vi "Add DefinedName.vi"(7 "Sheet Name":string, 8 "error in":errorcluster, 9 "Cell Range":string, 10 "Identifier":string, 11 "SpreadsheetDoc in":refnum<k24>) -> (0 "error out":errorcluster, 3 "SpreadsheetDoc out":refnum<k24>)   [LabVIEW 2019, in "Open Xml.lvlib"]
uses:
  Open Xml.lvlib
  D:/git/Open-Xml-LabVIEW/Source/DocumentFormat.OpenXml.dll
  DocumentFormat.OpenXml.dll
  D:/git/Open-Xml-LabVIEW/Source/DocumentFormat.OpenXml.Framework.dll
  DocumentFormat.OpenXml.Framework.dll
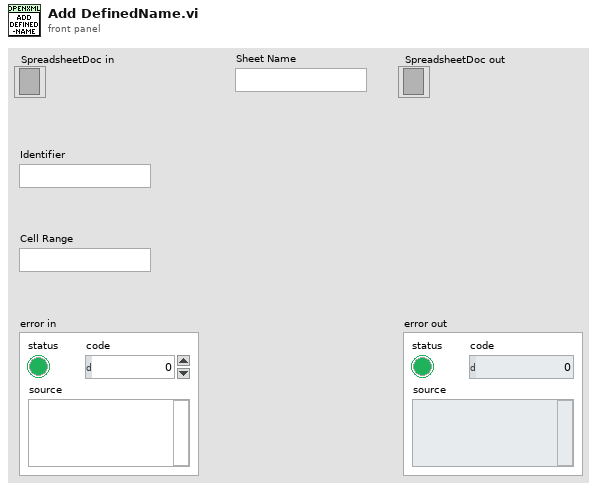
[diagram p1: front panel]
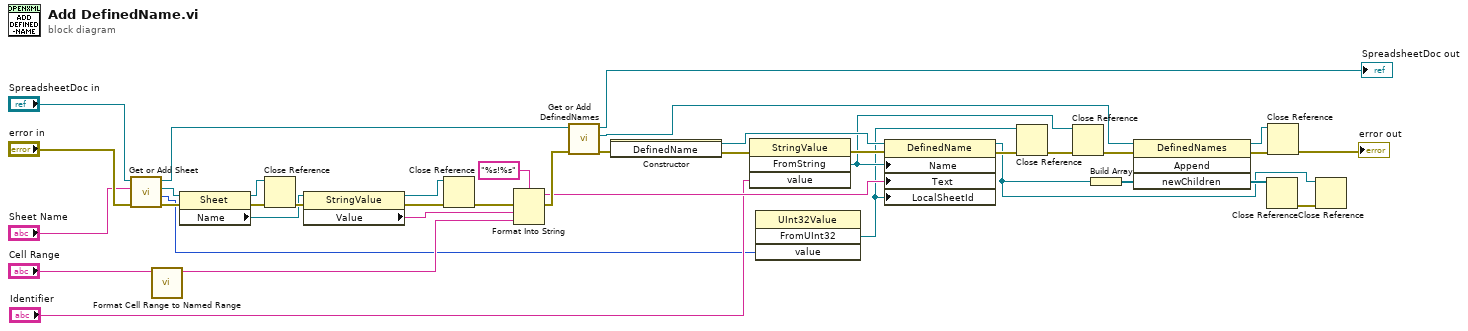
[diagram p0: block diagram]
diagram:
  n1 = call "Get or Add Sheet.vi"("error in"="error in", "Sheet Name"="Sheet Name", "SpreadsheetDoc in"="SpreadsheetDoc in") -> ("error out"=w10:errorcluster, "Sheet Index"=w2:i32, "Sheet"=w13:refnum<k24>, "SpreadsheetDoc out"=w16:refnum<k24>)  [unwired: 5 in]
  n2 = call "Format Cell Range to Named Range.vi"("Cell Range"="Cell Range") -> ("Formatted Cell Range"=w8:string)  [unwired: 10 in]
  n3 = property class="Sheet"(reference=w13, error in=w10) -> (reference out=w11:refnum<k24>, error out=w14:errorcluster, "Name"=w6:refnum<k24>)
  n4 = Close Reference(reference=w11, error in (no error)=w14) -> (error out=w12:errorcluster)
  n5 = property class="StringValue"(reference=w6, error in=w12) -> (reference out=w3:refnum<k24>, error out=w7:errorcluster, "Value"=w5:string)
  n6 = Close Reference(reference=w3, error in (no error)=w7) -> (error out=w4:errorcluster)
  n7 = Format Into String(format string="%s!%s", error in=w4, w5, w8) -> (resulting string=w23:string, error out=w25:errorcluster)  [unwired: 1 in]
  n8 = call "Get or Add DefinedNames.vi"("error in"=w25, "SpreadsheetDoc in"=w16) -> ("error out"=w38:errorcluster, "DefinedNames"=w37:refnum<k24>, "SpreadsheetDoc out"=→"SpreadsheetDoc out":refnum<k24>)  [unwired: 7 in]
  n9 = constructor class="DefinedName"(error in=w38) -> (reference out=w39:refnum<k24>, error out=w22:errorcluster)  [unwired: 2 in, 1 out]
  n10 = invoke class="StringValue" method="FromString"(error in=w22, "value"="Identifier") -> (error out=w21:errorcluster, "FromString"=w18:refnum<k24>)  [unwired: 2 in, 2 out]
  n11 = invoke class="UInt32Value" method="FromUInt32"("value"=w2) -> ("FromUInt32"=w1:refnum<k24>)  [unwired: 3 in, 3 out]
  n12 = property class="DefinedName"(reference=w39, error in=w21, "Name"=w18, "Text"=w23, "LocalSheetId"=w1) -> (reference out=w29:refnum<k24>, error out=w35:errorcluster)
  n13 = Close Reference(reference=w1, error in (no error)=w35) -> (error out=w9:errorcluster)
  n14 = Close Reference(reference=w18, error in (no error)=w9) -> (error out=w19:errorcluster)
  n15 = Build Array(w29) -> (w34:refnum<k24>[])
  n16 = invoke class="DefinedNames" method="Append"(reference=w37, error in=w19, "newChildren"=w34) -> (reference out=w32:refnum<k24>, error out=w33:errorcluster, "newChildren"=w31:refnum<k24>[])  [unwired: 1 in, 1 out]
  n17 = Close Reference(reference=w31) -> (error out=w30:errorcluster)  [unwired: 1 in]
  n18 = Close Reference(reference=w32, error in (no error)=w33) -> (error out=→"error out":errorcluster)
  n19 = Close Reference(reference=w29, error in (no error)=w30) -> ()  [unwired: 1 out]
